vi "Read Config.vi"(11 "file (use dialog)":path) -> (0 "error out":errorcluster, 3 "Config":T2)   [LabVIEW 2020, in "Sensor General Class.lvclass"]
uses:
  Sensor General Class.lvclass
panel:
  out "States":T1(array[cluster])
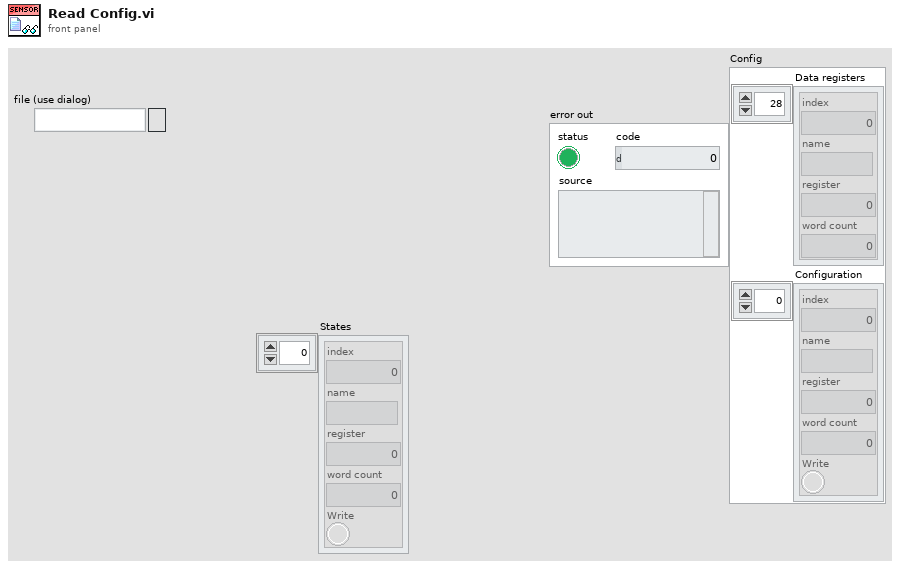
[diagram p1: front panel]
types:
  T1 = cluster{"index":i32, "name":string, "register":u16, "word count":u16, "Write":bool}[]
  T2 = cluster{"Data registers":cluster{"index":i32, "name":string, "register":u16, "word count":u16}[], "Configuration":cluster{"index":i32, "name":string, "register":u16, "word count":u16, "Write":bool}[]}
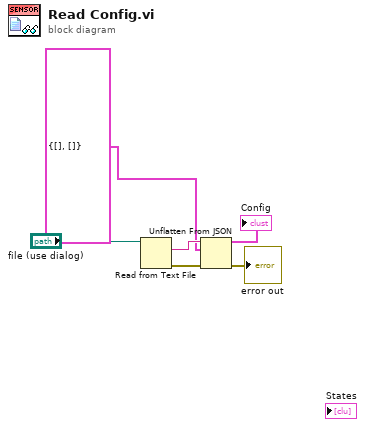
[diagram p0: block diagram]
diagram:
  n1 = Read from Text File(file (use dialog)="file (use dialog)") -> (text=w5:string, error out=w4:errorcluster)  [unwired: 3 in, 2 out]
  n2 = Unflatten From JSON(JSON string=w5, type and defaults=T2 {"Data registers"=[], "Configuration"=[]} ("output cluster"), error in (no error)=w4) -> (value=→"Config":T2, error out=→"error out":errorcluster)  [unwired: 4 in]
